vi "Acquire.vi"(8 "error in (no error)":errorcluster, 9 "Data Queue":refnum<queue>, 10 "Data Queue 2":refnum<queue>, 11 "Hardware Resources in":T1) -> (0 "error out":errorcluster, 3 "Hardware Resources out":T1)   [LabVIEW 2016, in "Acquisition.lvlib"]
doc: "Perform the acquisition. Replace the contents of this diagram with calls to acquisition hardware."
uses:
  Acquisition.lvlib
  Hardware Configuration.ctl
  <vilib>/DAQmx/read.llb/DAQmx Read (Analog 1D Wfm NChan NSamp).vi
  <vilib>/DAQmx/miscellaneous.llb/DAQmx Fill In Error Info.vi
  <resource>/objmgr/daqmx.rc
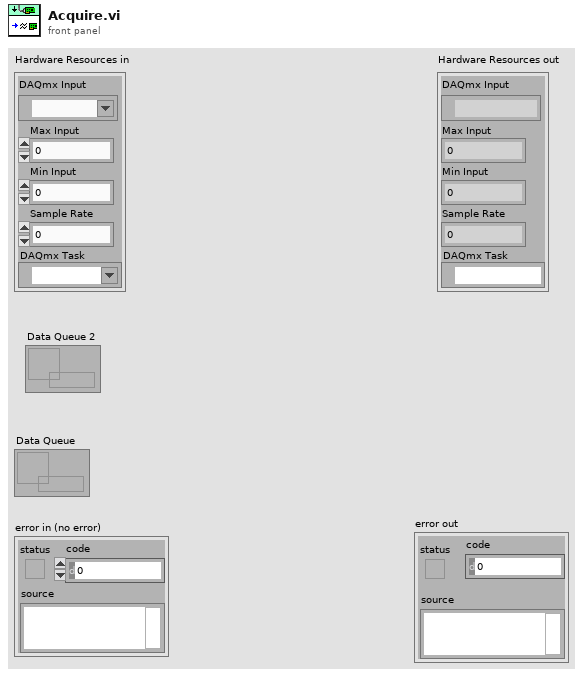
[diagram p1: front panel]
types:
  T1 = typedef "Acquisition.lvlib/Hardware Configuration.ctl" = cluster{"DAQmx Input":tag, "Max Input":dbl, "Min Input":dbl, "Sample Rate":dbl, "DAQmx Task":refnum<k21>}
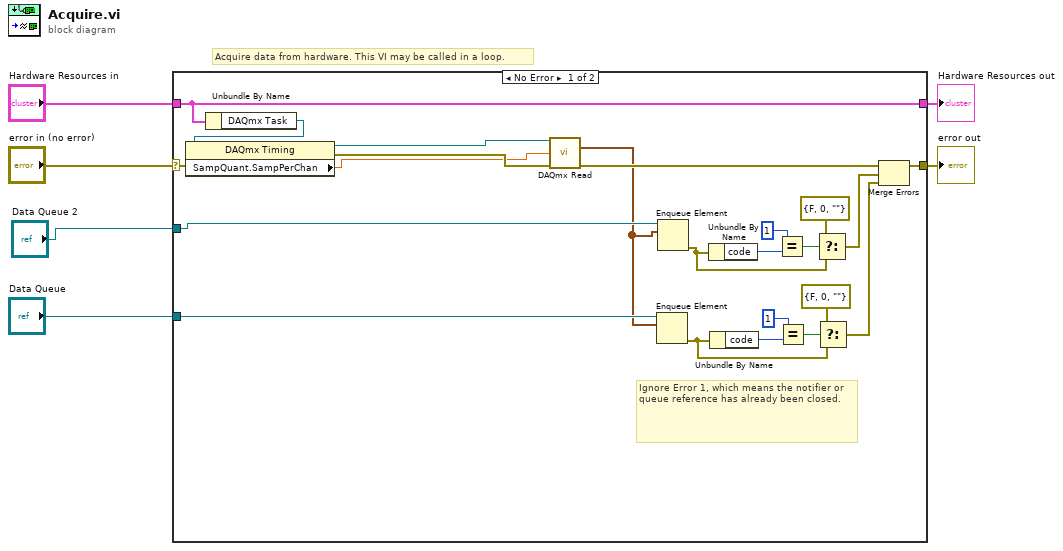
[diagram p0: block diagram]
diagram:
  # "Acquire data from hardware. This VI may be called in a loop."
  n1 = case shown="No Error" "error in (no error)" {
    selector: "error in (no error)" -> [w12 w30]
    tunnel: [w29 w30] -> w5
    tunnel: "Hardware Resources in" -> [w16 w31]
    tunnel: [w16 w31] -> w3
    tunnel: "Data Queue 2" -> [w9 _]
    tunnel: "Data Queue" -> [w17 _]
    frame No Error {
      # "Ignore Error 1, which means the notifier or queue reference has already been closed."
      n2 = Unbundle By Name(w16) -> ("DAQmx Task"=w14:refnum<k21>)
      n3 = property class="DAQmx Timing"(reference=w14, error in=w12) -> (reference out=w13:refnum<k21>, error out=w11:errorcluster, "SampQuant.SampPerChan"=w10:dbl)
      n4 = call-poly <vilib>:"DAQmx Read.vi"("task/channels in"=w13, "number of samples per channel"=w10, "error in"=w11) -> ("data"=w8:waveform(dbl)[], "error out"=w15:errorcluster)  [unwired: 10 in, 1 out]
      n5 = Enqueue Element(queue=w17, element=w8) -> (error out=w22:errorcluster)  [unwired: 2 in, 2 out]
      n6 = Enqueue Element(queue=w9, element=w8) -> (error out=w7:errorcluster)  [unwired: 2 in, 2 out]
      n7 = Unbundle By Name(w7) -> ("code"=w28:i32)
      n8 = Unbundle By Name(w22) -> ("code"=w19:i32)
      n9 = Equal?(x=1, y=w28) -> (x = y?=w26:bool)
      n10 = Equal?(x=1, y=w19) -> (x = y?=w21:bool)
      n11 = Select(t=errorcluster {"status"=FALSE, "code"=0, "source"=""} ("error constant"), s=w26, f=w7) -> (s? t:f=w25:errorcluster)
      n12 = Select(t=errorcluster {"status"=FALSE, "code"=0, "source"=""} ("error constant"), s=w21, f=w22) -> (s? t:f=w18:errorcluster)
      n13 = Merge Errors(w15, w25, w18) -> (w29:errorcluster)
    }
    frame Error {
    }
  }
  "Hardware Resources out" <- w3
  "error out" <- w5
